vi "Pfeiffer Vacuum HLT5xx Current State.vi"(8 "error in (no error)":errorcluster, 10 "Adress of unit":u16=1 min=1 max=999 step=1, 11 "COM Port Name in":refnum<visa-resource-name>="COM1") -> (0 "error out":errorcluster, 3 "response (data)":string)   [LabVIEW 2016]
doc: "This VI is an example of how to use the Pfeiffer Vacuum subVIs programmatically. This VI first initializes the instrument, takes measurements, then closes the instrument."
uses:
  Pfeiffer Vacuum.lvlib
panel:
  out "State out":u8(ring) items=["Init", "Preparing VacSYS", "Ready to Start", "Pumping", "--", "Stopping", "Calibrating", "Error", "Preparing MS", "Pumping internal TL", "Meas. Counter flow", "Meas. TwinFlow low", "Meas. TwinFlow high", "--", "--", "Meas. int. TL Counter flow", "Meas. int. TL TwinFlow low", "Meas. int. TL TwinFlow high", ""]
  # "Current State (read only)"
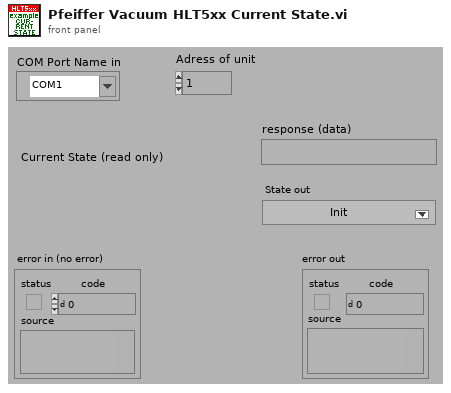
[diagram p1: front panel]
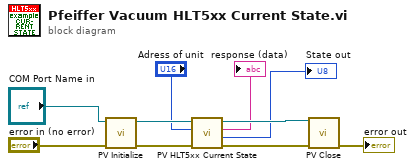
[diagram p0: block diagram]
diagram:
  n1 = call "PV Initialize.vi"("error in (no error)"="error in (no error)", "VISA session in"="COM Port Name in") -> ("error out"=w10:errorcluster, "VISA session out"=w8:refnum<visa-resource-name>)  [unwired: 8 in]
  n2 = call "PV HLT5xx Current State.vi"("error in (no error)"=w10, "Adress of unit"="Adress of unit", "VISA session"=w8) -> ("error out"=w9:errorcluster, "State out"=→"State out":u8, "response (data) out"=→"response (data)":string, "dup VISA session"=w7:refnum<visa-resource-name>)  [unwired: 5 in]
  n3 = call "PV Close.vi"("VISA session"=w7, "error in (no error)"=w9) -> ("error out"=→"error out":errorcluster)  [unwired: 13 in]
